vi "pl1000SetDo.vi"(8 "error in (no error)":errorcluster, 9 "DO Channel":i32, 10 "DO State":bool, 11 "pl1000 handle":i16) -> (0 "error out":errorcluster, 3 "pl1000 handle out":i16)   [LabVIEW 2010]
uses:
  pl1000.dll
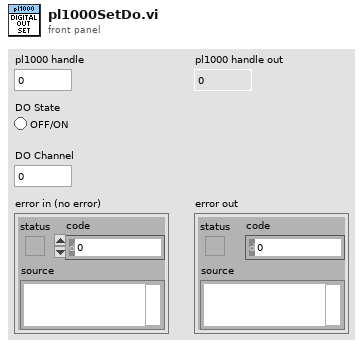
[diagram p1: front panel]
types:
  T1 = cluster{"status":bool, "code":u32, "source":string}
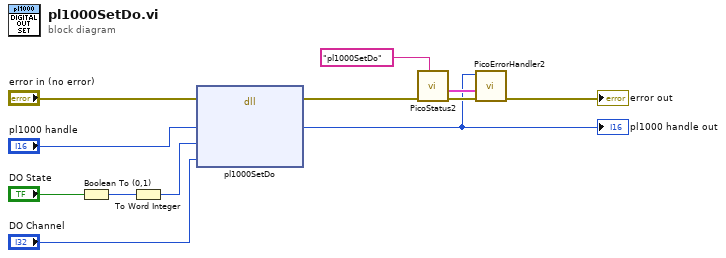
[diagram p0: block diagram]
diagram:
  n1 = Boolean To (0,1)(Boolean="DO State") -> (0, 1=w9:i16)
  n2 = To Word Integer(number=w9) -> (16bit integer=w8:i16)
  n3 = dll-call lib="pl1000.dll" fn="pl1000SetDo"(error in="error in (no error)", "handle"="pl1000 handle", "doValue"=w8, "doNo"="DO Channel") -> (error out=w3:errorcluster, "handle"=w2:i16)  [unwired: 5 in, 1 out]
  "pl1000 handle out" <- w2
  n4 = call "PicoStatus2.vi"("PICO source"="pl1000SetDo", "Error in"=w3) -> ("error out"=w6:errorcluster, "PICO_STATUS out"=w5:T1)  [unwired: 6 in]
  n5 = call "PicoErrorHandler2.vi"("error in (no error)"=w6, "PICO_STATUS in"=w5, "handle In"=w2) -> ("error out"=→"error out":errorcluster)  [unwired: 8 in]
